vi "pidInitializer.vi"(9 "error in":errorcluster, 10 "PIDF":cluster{"P":dbl, "I":dbl, "D":dbl, "F":dbl} {"F" format="%#_13g"; "D" format="%#_13g"; "I" format="%#_13g"; "P" format="%#_13g"}, 11 "Can IDs":T7) -> (2 "error out":errorcluster, 3 "Motors":T6)   [LabVIEW 2020]
uses:
  <vilib>/Rock Robotics/WPI/MotorControl/WPI_MotorControlDeviceRef.ctl
  <vilib>/Rock Robotics/WPI/MotorControl/WPI_MotorControlType.ctl
  <vilib>/Rock Robotics/SystemInterfaces/DIO/FPGA_DIOPWMChannel.ctl
  <vilib>/Rock Robotics/WPI/PWM/WPI_PWMDeadband.ctl
  <vilib>/Rock Robotics/SystemInterfaces/DIO/FPGA_DIOChannel.ctl
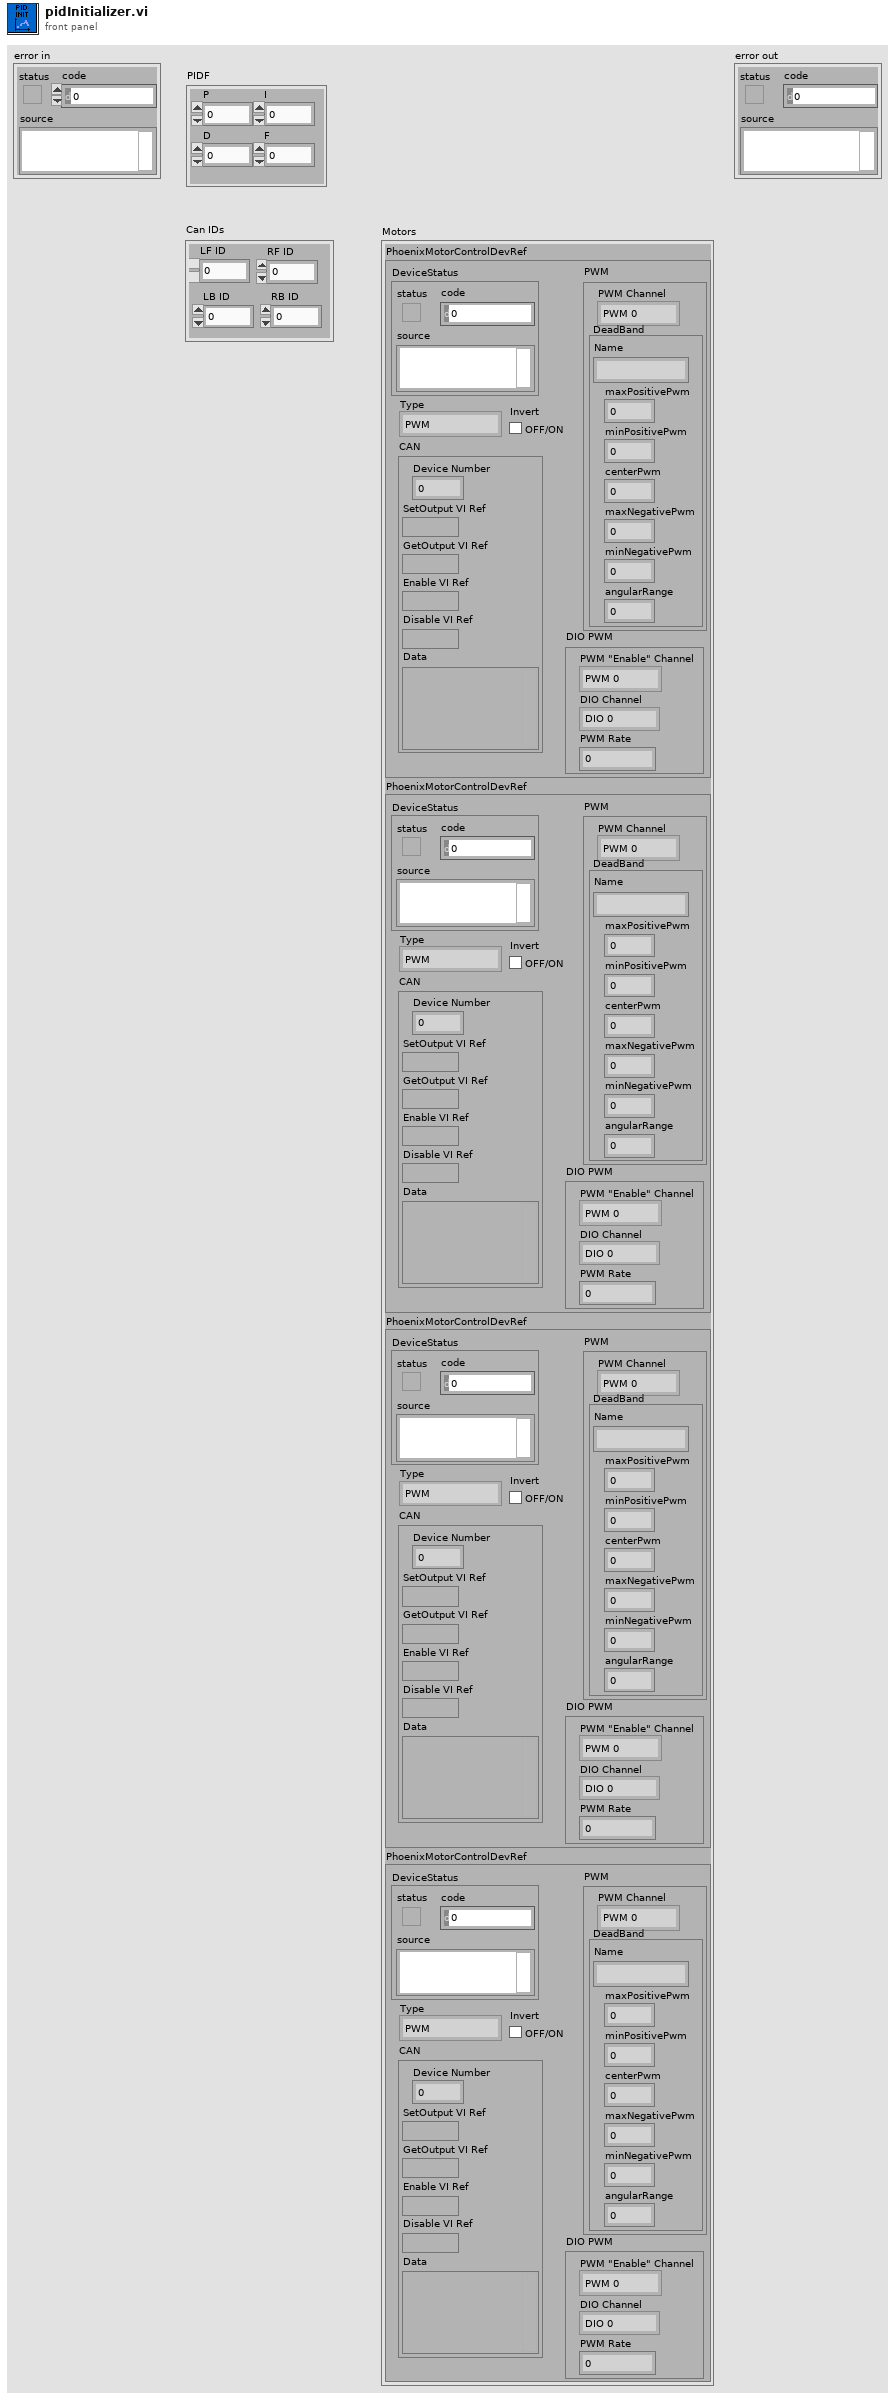
[diagram p1: front panel]
types:
  T1 = typedef "WPI_MotorControlDeviceRef.ctl" = cluster{"DeviceStatus":errorcluster, "Type":T2, "PWM":cluster{"PWM Channel":T3, "DeadBand":T4}, "CAN":cluster{"Device Number":u8, "SetOutput VI Ref":variant, "GetOutput VI Ref":variant, "Enable VI Ref":variant, "Disable VI Ref":variant, "Data":variant}, "Invert":bool, "DIO PWM":cluster{"PWM \"Enable\" Channel":T3, "DIOChannel":T5, "PWM Rate":dbl}}
  T2 = typedef "WPI_MotorControlType.ctl" = enum16{"PWM", "CAN", "DIO PWM"}
  T3 = typedef "FPGA_DIOPWMChannel.ctl" = enum8{"PWM 0", "PWM 1", "PWM 2", "PWM 3", "PWM 4", "PWM 5", "PWM 6", "PWM 7", "PWM 8", "PWM 9", "PWM MXP 0", "PWM MXP 1", "PWM MXP 2", "PWM MXP 3", "PWM MXP 4", "PWM MXP 5", "PWM MXP 6", "PWM MXP 7", "PWM MXP 8", "PWM MXP 9", "Invalid"}
  T4 = typedef "WPI_PWMDeadband.ctl" = cluster{"Name":string, "maxPositivePwm":i32, "minPositivePwm":i32, "centerPwm":i32, "maxNegativePwm":i32, "minNegativePwm":i32, "angularRange":u16}
  T5 = typedef "FPGA_DIOChannel.ctl" = enum8{"DIO 0", "DIO 1", "DIO 2", "DIO 3", "DIO 4", "DIO 5", "DIO 6", "DIO 7", "DIO 8", "DIO 9", "DIO MXP 0", "DIO MXP 1", "DIO MXP 2", "DIO MXP 3", "DIO MXP 4", "DIO MXP 5", "DIO MXP 6", "DIO MXP 7", "DIO MXP 8", "DIO MXP 9", "DIO MXP 10", "DIO MXP 11", "DIO MXP 12", "DIO MXP 13", "DIO MXP 14", "DIO MXP 15", "SPI Port CS1", "SPI Port CS2", "SPI Port CS3", "SPI Port MISO", "SPI Port MOSI", "Invalid"}
  T6 = cluster{"PhoenixMotorControlDevRef":T1, "PhoenixMotorControlDevRef":T1, "PhoenixMotorControlDevRef":T1, "PhoenixMotorControlDevRef":T1}
  T7 = cluster{"LF ID":u8, "LB ID":u8, "RF ID":u8, "RB ID":u8}
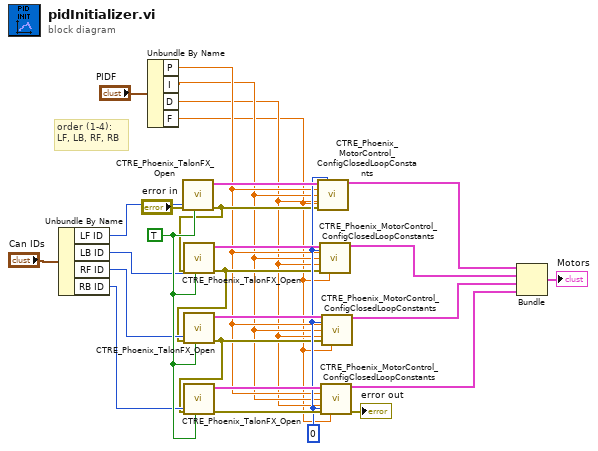
[diagram p0: block diagram]
diagram:
  w21 = 0 ("slotIdx")
  w22 = TRUE ("Invert")
  # "order (1-4):\nLF, LB, RF, RB"
  n1 = Unbundle By Name("Can IDs") -> ("LF ID"=w19:u8, "LB ID"=w18:u8, "RF ID"=w17:u8, "RB ID"=w16:u8)
  n2 = Unbundle By Name("PIDF") -> ("P"=w6:dbl, "I"=w5:dbl, "D"=w4:dbl, "F"=w3:dbl)
  n3 = call <vilib>:"CTRE_Phoenix_TalonFX_Open.vi"("Invert"=w22, "error in"="error in", "Device Number"=w19) -> ("error out"=w10:errorcluster, "PhoenixMotorControlDevRef"=w27:T1)  [unwired: 7 in]
  n4 = call <vilib>:"CTRE_Phoenix_TalonFX_Open.vi"("Invert"=w22, "error in"=w10, "Device Number"=w18) -> ("error out"=w9:errorcluster, "PhoenixMotorControlDevRef"=w26:T1)  [unwired: 7 in]
  n5 = call <vilib>:"CTRE_Phoenix_TalonFX_Open.vi"("Invert"=w22, "error in"=w9, "Device Number"=w17) -> ("error out"=w8:errorcluster, "PhoenixMotorControlDevRef"=w25:T1)  [unwired: 7 in]
  n6 = call <vilib>:"CTRE_Phoenix_TalonFX_Open.vi"("Invert"=w22, "error in"=w8, "Device Number"=w16) -> ("error out"=w23:errorcluster, "PhoenixMotorControlDevRef"=w24:T1)  [unwired: 7 in]
  n7 = call <vilib>:"CTRE_Phoenix_MotorControl_ConfigClosedLoopConstants.vi"("PhoenixMotorControlDevRef"=w27, "slotIdx"=w21, "P"=w6, "I"=w5, "D"=w4, "error in (no error)"=w10, "F"=w3) -> ("PhoenixMotorControlDevRef"=w15:T1)  [unwired: 7 in, 1 out]
  n8 = call <vilib>:"CTRE_Phoenix_MotorControl_ConfigClosedLoopConstants.vi"("PhoenixMotorControlDevRef"=w26, "slotIdx"=w21, "P"=w6, "I"=w5, "D"=w4, "error in (no error)"=w9, "F"=w3) -> ("PhoenixMotorControlDevRef"=w14:T1)  [unwired: 7 in, 1 out]
  n9 = call <vilib>:"CTRE_Phoenix_MotorControl_ConfigClosedLoopConstants.vi"("PhoenixMotorControlDevRef"=w24, "slotIdx"=w21, "P"=w6, "I"=w5, "D"=w4, "error in (no error)"=w23, "F"=w3) -> ("PhoenixMotorControlDevRef"=w12:T1, "error out"=→"error out":errorcluster)  [unwired: 7 in]
  n10 = call <vilib>:"CTRE_Phoenix_MotorControl_ConfigClosedLoopConstants.vi"("PhoenixMotorControlDevRef"=w25, "slotIdx"=w21, "P"=w6, "I"=w5, "D"=w4, "error in (no error)"=w8, "F"=w3) -> ("PhoenixMotorControlDevRef"=w13:T1)  [unwired: 7 in, 1 out]
  n11 = Bundle("PhoenixMotorControlDevRef"=w15, "PhoenixMotorControlDevRef"=w14, "PhoenixMotorControlDevRef"=w13, "PhoenixMotorControlDevRef"=w12) -> (→"Motors":T6)  [unwired: 1 in]
